vi "To String.vi"(8 "error in (no error)":errorcluster, 11 "Is Stringifiable in":refnum<class "Is Stringifiable.lvclass">) -> (0 "error out":errorcluster, 2 "string":string, 3 "Is Stringifiable out":refnum<class "Is Stringifiable.lvclass">)   [LabVIEW 2020, in "PV Access.lvlib" / "PV Data.lvlib" / "Is Stringifiable.lvclass"]
uses:
  Is Stringifiable.lvclass
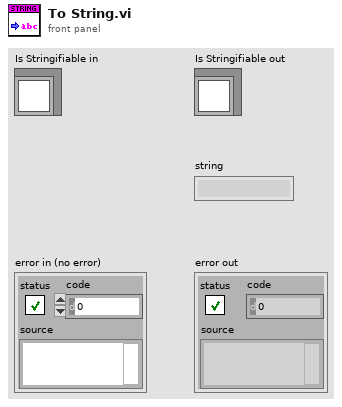
[diagram p1: front panel]
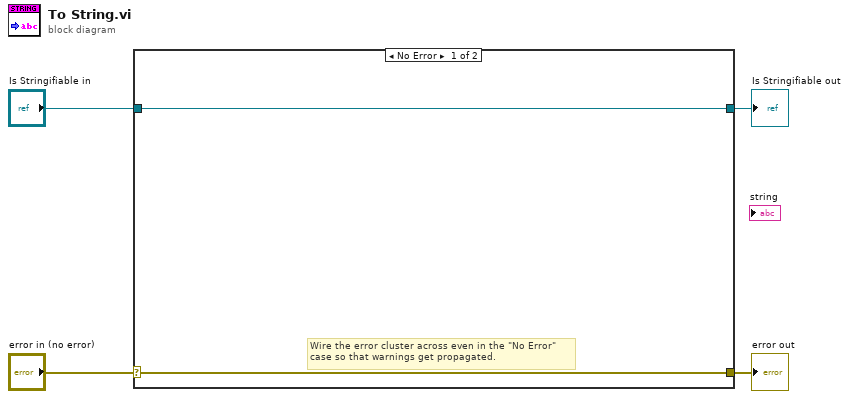
[diagram p0: block diagram]
diagram:
  n1 = case shown="No Error" "error in (no error)" {
    selector: "error in (no error)" -> [w5 w8]
    tunnel: [w5 w8] -> w3
    tunnel: [w6 w7] -> w1
    tunnel: "Is Stringifiable in" -> [w6 w7]
    frame No Error {
      # "Wire the error cluster across even in the \"No Error\"\ncase so that warnings get propagated."
    }
    frame Error {
    }
  }
  "error out" <- w3
  "Is Stringifiable out" <- w1
